vi "Gear Controller.vi"(8 "error in":errorcluster) -> ()   [LabVIEW 2016]
doc: "This VI executes continuously carrying out the current operation and responding to updates or new operations. It will often contain the timing or control code that is difficult to place directly in TeleOp. This VI generally opens all sensors and motors and isolates the rest of the robot code from knowing how the operations are carried out."
uses:
  Gear Operations.ctl
  Gear Setpoints.ctl
  <vilib>/Rock Robotics/WPI/Solenoid/WPI_SolenoidSetEnum.vi
  <vilib>/Rock Robotics/WPI/Solenoid/WPI_SolenoidValue.ctl
  <vilib>/Rock Robotics/Network Tables/NT Write Boolean.vi
panel:
  out "Current\nCmd":string="Started at  Mon 20 Feb 2017 09:37:39 PM CST\nDefault: Reserve,  S 0.0, D 0.000000"
  # "Tip: It may be helpful to observe inputs and sensor values.\nYou may also want to display tuning or debugging controls."
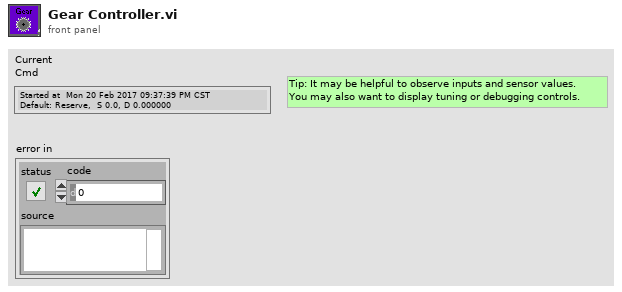
[diagram p1: front panel]
types:
  T1 = typedef "Gear Setpoints.ctl" = cluster{"Operation":T2, "Setpoint":dbl, "Duration":dbl}
  T2 = typedef "Gear Operations.ctl" = enum16{"Reserve", "Read Current", "Immediate", "Go to Scoring", "Go to Intake", "Arms out", "Spin rollers", "Arms in"}
  T3 = typedef "Command Status Info.ctl" = cluster{"Name":string, "Status":T4, "notifier out":T5}
  T4 = typedef "Completion Status.ctl" = enum16{"Successful", "Aborted", "Incomplete"}
  T5 = typedef "Completion Notifier.ctl" = refnum<notifier>
  T6 = cluster{"Default Command":T1, "Command Timing":cluster{"Start Time (ms)":u32, "Iterations":i32}, "Command Arguments":cluster{"Command Info":T3, "Description":string, "Default Command":T1, "notifier out":refnum<notifier>, "Subsystem Name":string}}
  T7 = typedef "WPI_SolenoidValue.ctl" = enum16{"Off", "On", "Forward", "Reverse"}
  T8 = typedef "WPI_DriverStationRobotMode2.ctl" = enum16{"Autonomous Disabled", "Autonomous Enabled", "Teleop Disabled", "Teleop Enabled", "Disconnected", "Finish", "Test Disabled", "Test Enabled", "Emergency Stopped"}
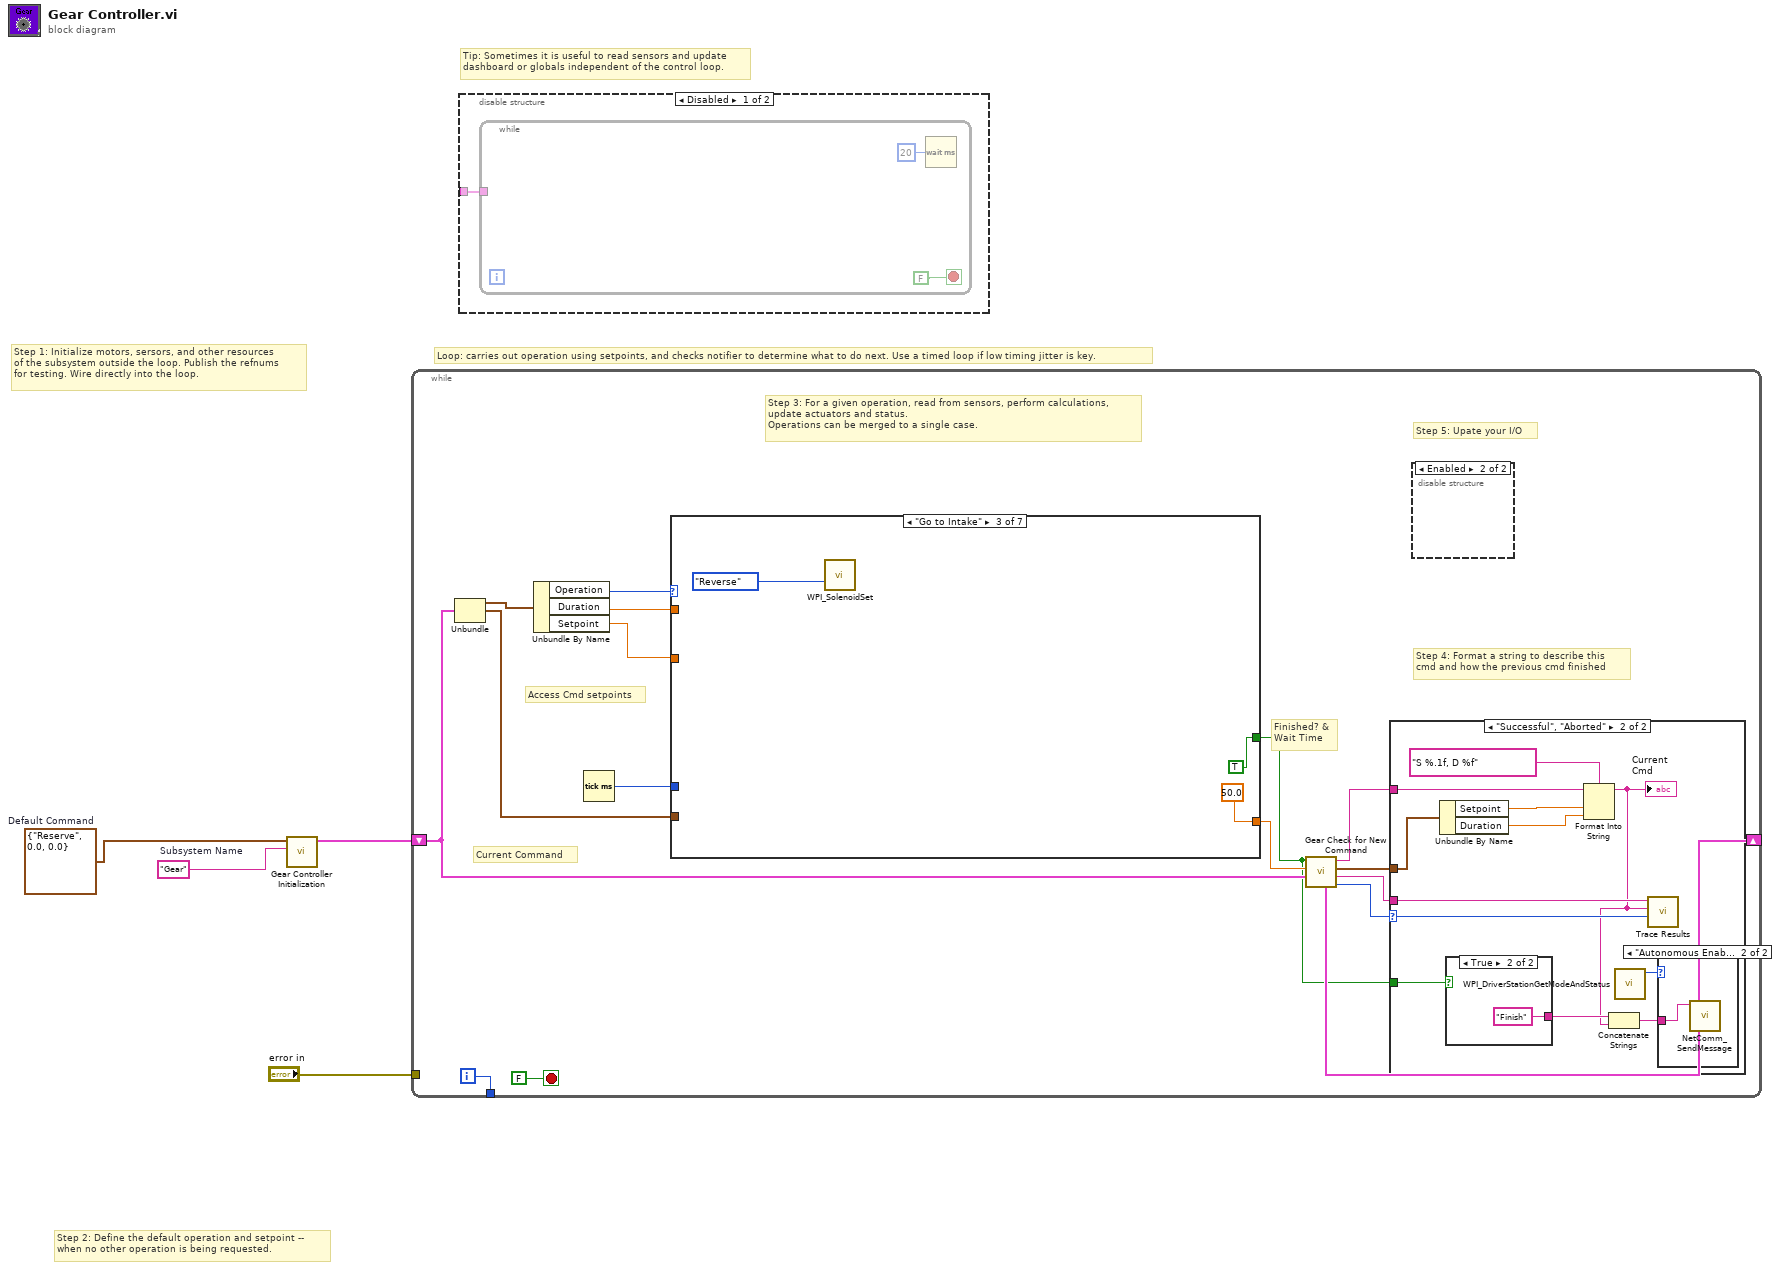
[diagram p0: block diagram]
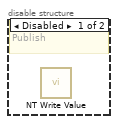
[diagram p3: hidden frame]
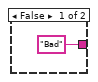
[diagram p5: hidden frame]
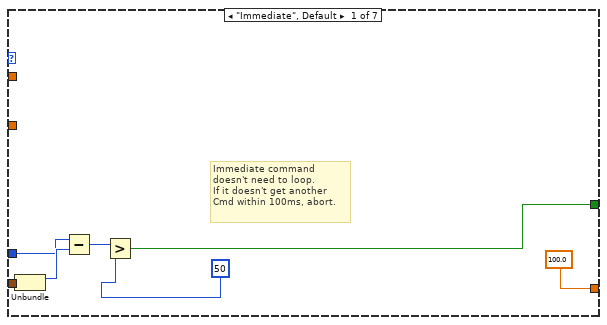
[diagram p7: hidden frame]
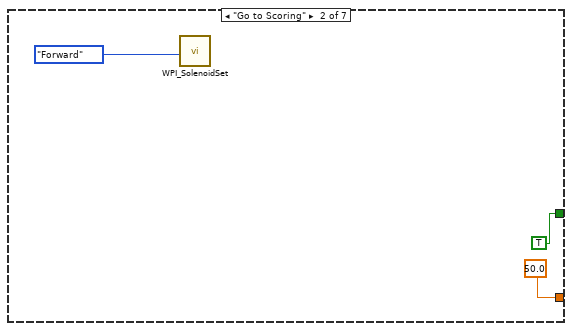
[diagram p8: hidden frame]
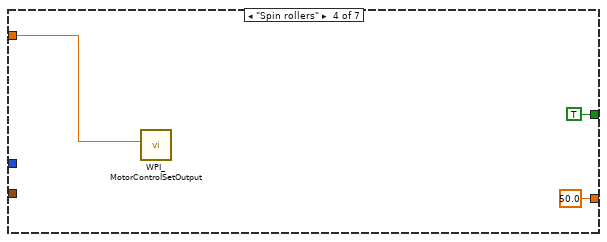
[diagram p9: hidden frame]
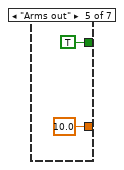
[diagram p10: hidden frame]
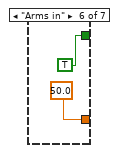
[diagram p11: hidden frame]
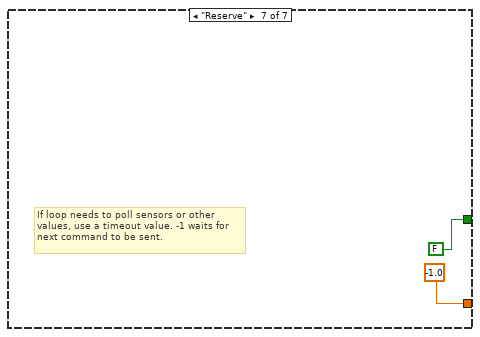
[diagram p12: hidden frame]
diagram:
  w1 = T1 {"Operation"=enum."Reserve", "Setpoint"=0.0, "Duration"=0.0}  # Default Command
  w2 = "Gear"  # Subsystem Name
  # "Tip: Sometimes it is useful to read sensors and update\ndashboard or globals independent of the control loop."
  # "Step 2: Define the default operation and setpoint --\nwhen no other operation is being requested."
  # "Step 1: Initialize motors, sersors, and other resources\nof the subsystem outside the loop. Publish the refnums\nfor testing. Wire directly into the loop."
  # "Loop: carries out operation using setpoints, and checks notifier to determine what to do next. Use a timed loop if low timing jitter is key."
  n1 = call "Gear Controller Initialization.vi"("Subsystem Name"=w2, "Default Command"=w1) -> ("Command Info"=w3:T6)  [unwired: 9 in]
  n2 = while {
    shift-right: [w11] -> _
    shift-left: w3 -> [w12]
    tunnel: [w19] -> _
    tunnel: "error in" -> [_]
    i -> [w19]
    stop <- FALSE stop-if-true
    # "Step 5: Upate your I/O"
    # "Step 4: Format a string to describe this\ncmd and how the previous cmd finished"
    # "Current Command"
    # "Access Cmd setpoints"
    # "Finished? &\nWait Time"
    # "Step 3: For a given operation, read from sensors, perform calculations,\nupdate actuators and status.\nOperations can be merged to a single case."
    n3 = Unbundle(w12) -> ("Default Command"=w18:T1, "Command Timing"=w14:cluster{"Start Time (ms)":u32, "Iterations":i32})  [unwired: 1 out]
    n4 = Unbundle By Name(w18) -> ("Operation"=w17:T2, "Duration"=w16:dbl, "Setpoint"=w13:dbl)
    n5 = Tick Count (ms)() -> (millisecond timer value=w15:u32)
    n6 = case shown="\"Go to Intake\"" w17 {
      tunnel: [100.0 50.0 50.0 50.0 10.0 50.0 -1.0] -> w10
      tunnel: [w36 TRUE ("ignore previous (F)") TRUE ("ignore previous (F)") TRUE ("ignore previous (F)") TRUE ("ignore previous (F)") TRUE ("ignore previous (F)") FALSE ("ignore previous (F)")] -> w5
      tunnel: w14 -> [w38 _ _ _ _ _ _]
      tunnel: w16 -> [_ _ _ _ _ _ _]
      tunnel: w15 -> [w37 _ _ _ _ _ _]
      tunnel: w13 -> [_ _ _ w51 _ _ _]
      frame "Immediate", Default {
        # "Immediate command\ndoesn't need to loop.\nIf it doesn't get another\nCmd within 100ms, abort."
        n7 = Unbundle(w38) -> ("Start Time (ms)"=w41:u32)  [unwired: 1 out]
        n8 = Subtract(x=w37, y=w41) -> (x-y=w40:u32)
        n9 = Greater?(x=w40, y=u8 50 ("Left Motor")) -> (0:w36:bool)
      }
      frame "Go to Scoring" {
        n10 = call-poly <vilib>:"WPI_SolenoidSet.vi"("Value"=WPI_SolenoidValue."Forward") -> ()  [unwired: 9 in, 2 out]
      }
      frame "Go to Intake" {
        n11 = call-poly <vilib>:"WPI_SolenoidSet.vi"("Value"=WPI_SolenoidValue."Reverse") -> ()  [unwired: 9 in, 2 out]
      }
      frame "Spin rollers" {
        n12 = call <vilib>:"WPI_MotorControlSetOutput.vi"("Output"=w51) -> ()  [unwired: 8 in, 3 out]
      }
      frame "Arms out" {
      }
      frame "Arms in" {
      }
      frame "Reserve" {
        # "If loop needs to poll sensors or other\nvalues, use a timeout value. -1 waits for\nnext command to be sent."
      }
    }
    n13 = call "Gear Check for New Command.vi"("Current Command"=w12, "Wait time (ms)"=w10, "Finished?"=w5) -> ("Completion"=w6:T4, "Subsystem Name"=w7:string, "Current Command"=w8:T1, "Initial Trace String"=w9:string, "NextCommand"=w11:T6)  [unwired: 4 in]
    n14 = case shown="\"Successful\", \"Aborted\"" w6 {
      selector: w6 -> [_ w32]
      tunnel: w9 -> [_ w28]
      tunnel: w8 -> [_ w29]
      tunnel: w7 -> [_ w26]
      tunnel: w5 -> [_ w22]
      frame "Incomplete", Default {
        # "Continuing current command"
      }
      frame "Successful", "Aborted" {
        # "Report and setup for next command"
        n15 = Unbundle By Name(w29) -> ("Setpoint"=w31:dbl, "Duration"=w27:dbl)
        n16 = case shown="True" w22 {
          tunnel: ["Bad" "Finish"] -> w24
          frame False {
          }
          frame True {
          }
        }
        n17 = Format Into String(format string="S %.1f, D %f", initial string=w28, w31, w27) -> (resulting string=w21:string)  [unwired: 1 in, 1 out]
        "Current\nCmd" <- w21
        n18 = Concatenate Strings(w24, w21) -> (w23:string)
        n19 = call <vilib>:"WPI_DriverStationGetModeAndStatus.vi"() -> ("Robot Mode"=w25:T8)  [unwired: 10 in, 1 out]
        n20 = call <vilib>:"Trace Results.vi"("Status of previous command"=w32, "Description"=w21, "Subsystem"=w26) -> ()  [unwired: 9 in]
        n21 = case shown="\"Autonomous Enabled\"" w25 {
          tunnel: w23 -> [_ w35]
          frame "Autonomous Disabled", Default {
          }
          frame "Autonomous Enabled" {
            n22 = call <vilib>:"NetComm_SendMessage.vi"("Message"=w35) -> ()  [unwired: 11 in]
          }
        }
      }
    }
    n23 = disable-structure shown="Enabled" {
      frame Disabled {
        # "Publish"
        n24 = call-poly <vilib>:"NT Write Value.vi"() -> ()  [unwired: 11 in, 1 out]
      }
      frame Enabled {
      }
    }
  }
  n25 = disable-structure shown="Disabled" {
    disable-tunnel: _ -> [w58 _]
    frame Disabled {
      n26 = while {
        tunnel: w58 -> [_]
        stop <- FALSE stop-if-true
        n27 = Wait (ms)(milliseconds to wait=u32 20) -> ()  [unwired: 1 out]
      }
    }
    frame Enabled {
    }
  }
